vi "PH_ImageCoG_Plotter.ProcCases.vi"(0 "i ref in":refnum<vi>, 1 "selector":string, 2 "data":T1, 3 "call cluster":T2={"Object"="", "Selector"="", "CallType"=enum."synchronous", "Async Object"="", "Async Selector"="", "Data Descriptor"="", "Data"=[], "Error #"=0, "Expire"=0}, 5 "error in":errorcluster) -> (14 "i ref out":refnum<vi>, 17 "answer cluster":T2={"Object"="", "Selector"="", "CallType"=enum."synchronous", "Async Object"="", "Async Selector"="", "Data Descriptor"="", "Data"=[], "Error #"=0, "Expire"=0}, 19 "error out":errorcluster)   [LabVIEW 2014, in "PH_ImageCoG_Plotter.lvlib"]
doc: "This method is called by a process from within the default case in the event loop. The methods of a class that are linked to events will be called from THIS method. Add your code here."
uses:
  PH_ImageCoG_Plotter.lvlib
  CS_Core/CSSystem/CoreDefs/CoreDefs.call_type.ctl
  CS_Core/BaseProcess/BaseProcess.descriptor string definition.ctl
  CS_Core/CSSystem/CoreDefs/CoreDefs.rawDataType.ctl
  CS_Core/CSSystem/CoreLib/CoreLib.byte array 2 int.vi
  CS_Core/CSSystem/CoreLib/CoreLib.string 2 byte array.vi
  CS_Core/CSSystem/CoreLib/CoreLib.byte array 2 short.vi
  CS_Core/CSSystem/CoreLib/CoreLib.byte array 2 string.vi
  CS_Core/CSSystem/CoreLib/CoreLib.lvlib
  CS_Core/BaseProcess/BaseProcess.lvlib
  CS_Core/CAEObj/CAEObj.lvlib
  PH_Basics/PH_Img_BaseClass/PH_Img_BaseClass.lvlib
  PH_Basics/PH_Cam_BaseClass/PH_Cam_BaseClass.lvlib
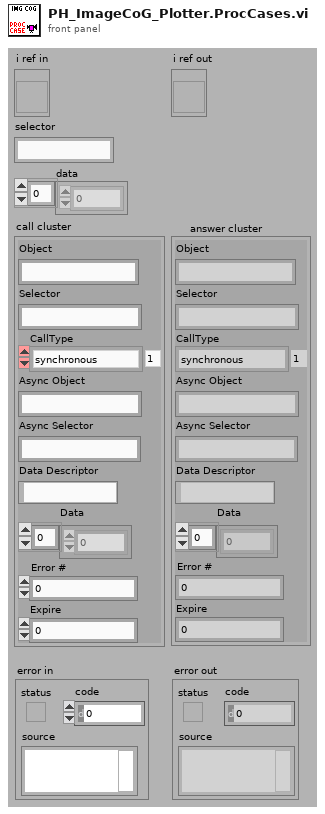
[diagram p1: front panel]
types:
  T1 = typedef "CoreDefs.rawDataType.ctl" = i8[]
  T2 = typedef "CoreDefs.call_type.ctl" = cluster{"Object":string, "Selector":string, "CallType":enum16{"simple", "synchronous", "asynchronous"}, "Async Object":string, "Async Selector":string, "Data Descriptor":T3, "Data":T1, "Error #":i32, "Expire":u32}
  T3 = typedef "BaseProcess.lvlib/BaseProcess.descriptor string definition.ctl" = string
  T4 = typedef "PH_ImageCoG_Plotter.lvlib/PH_ImageCoG_Plotter.i attribute.ctl" = cluster{"GUI Refs":cluster{"Delete":refnum<vi>, "Calibration status":refnum<vi>, "BI subtracted":refnum<vi>, "calc Beam Anal":refnum<vi>, "CoG - x":refnum<vi>, "CoG - y":refnum<vi>, "Type":refnum<vi>, "Center":refnum<vi>, "exp - X":refnum<vi>, "exp - Y":refnum<vi>, "Delta - X":refnum<vi>, "Delta - Y":refnum<vi>, "Available Cams":refnum<vi>, "CoG X":refnum<vi>, "CoG Y":refnum<vi>, "Delta X":refnum<vi>, "Delta Y":refnum<vi>, "Export Data":refnum<vi>, "Calibration data":refnum<vi>}, "Calibration":cluster{"Status":T5, "Calibration data":T6, "Calibration Data File":path}, "Beam Analysis":cluster{"on":bool, "exp - X":i32, "exp - Y":i32, "Type":bool, "Data":cluster{"current time":timestamp, "CoG-x":dbl, "CoG-y":dbl, "Delta-x":dbl, "Delta-y":dbl}[], "Datasets strored":i32, "Dataarray Size":i32}, "Cam instances":string[], "DIM Service Events":T7[], "Images":cluster{"Background":T9, "OP":T9, "GUI":T9}}
  T5 = typedef "PH_StatusHandler.lvlib/PH_StatusHandler.Status.ctl" = i16
  T6 = typedef "PH_ImageCalibrator.lvlib/PH_ImageCalibrator.Calibration Data.ctl" = cluster{"Date":string, "Time":string, "Cam Settings":cluster{"Cam ID":string, "Gain":dbl, "Brightness":dbl, "Shutter":dbl, "Cam Error":bool, "Mode":i32}, "Background Image":cluster{"Image":dbl[][], "Image Error":bool}, "Linear Calibration":cluster{"Calibration Factor":dbl, "not mm or mrad":bool}, "Energy Calibration":cluster{"Calibration Factor":dbl, "no mJ":bool}}
  T7 = typedef "BaseProcess.lvlib/BaseProcess.event definition.ctl" = cluster{"CAEEvtDef":T8, "Data Descriptor":T3}
  T8 = typedef "CAEObj.lvlib/CAEObj.event definition.ctl" = cluster{"URL":string, "enable":bool, "ignoreResID":bool}
  T9 = typedef "IMAQ Image.ctl" = refnum<image>
  T10 = typedef "PH_Cam_BaseClass.lvlib/PH_Cam_BaseClass.Settings.ctl" = cluster{"Cam ID":string, "Gain":dbl, "Brightness":dbl, "Shutter":dbl, "Mode":i32}
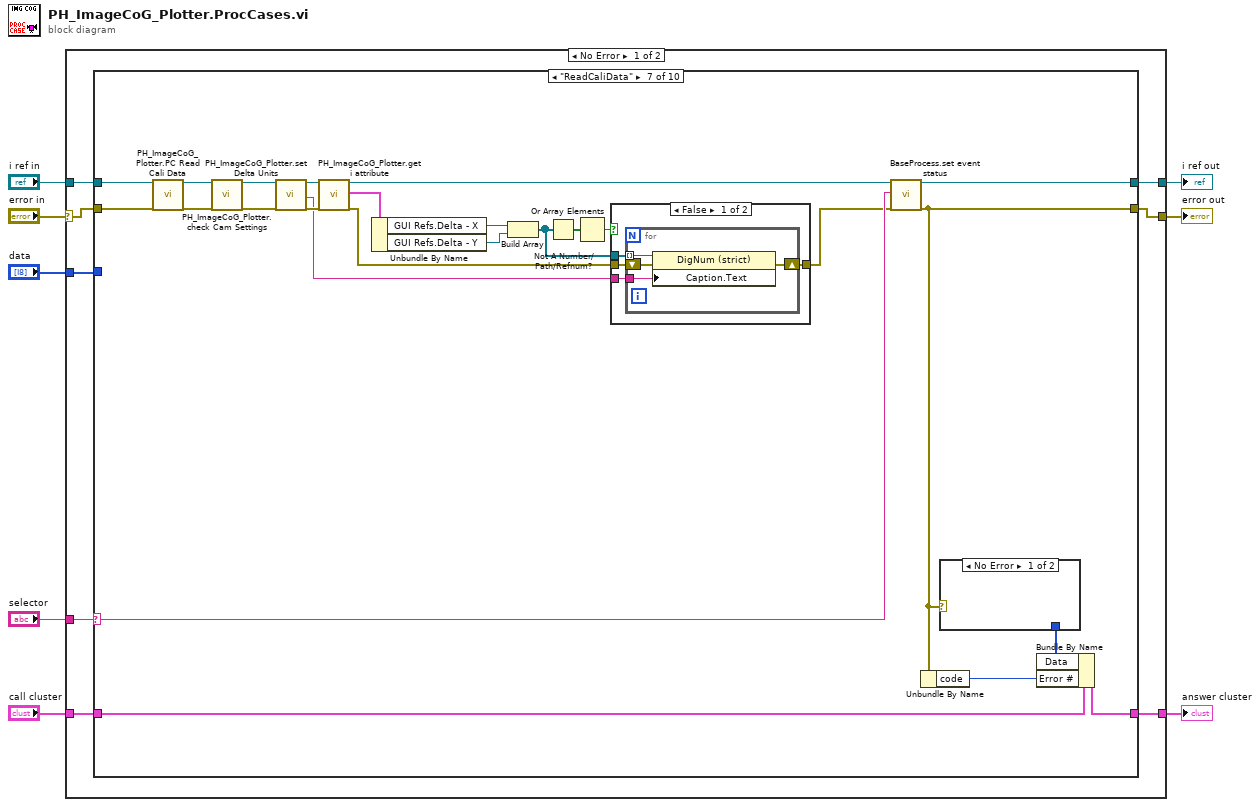
[diagram p0: block diagram]
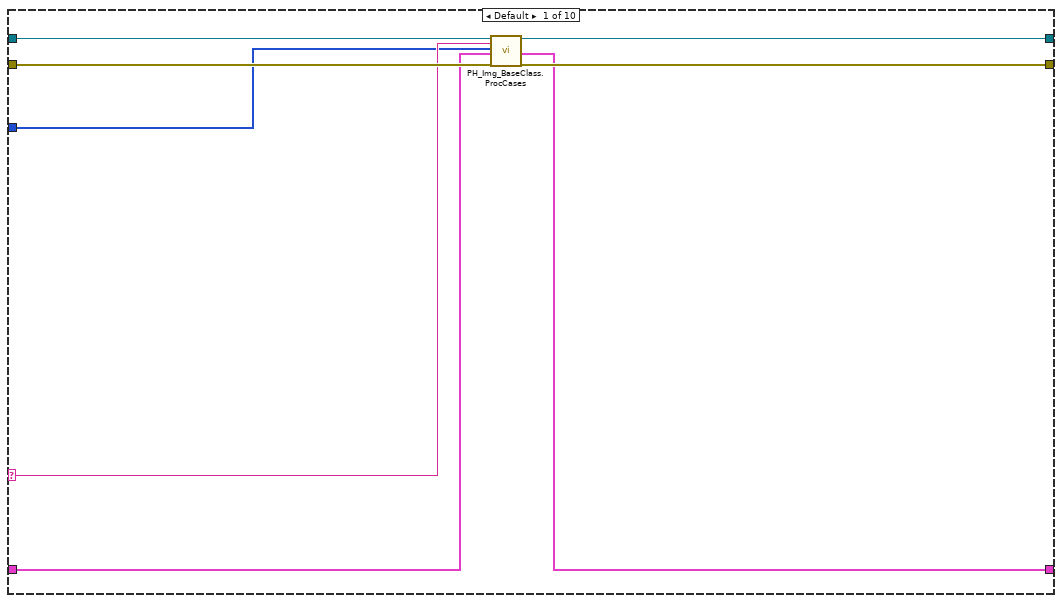
[diagram p2: hidden frame]
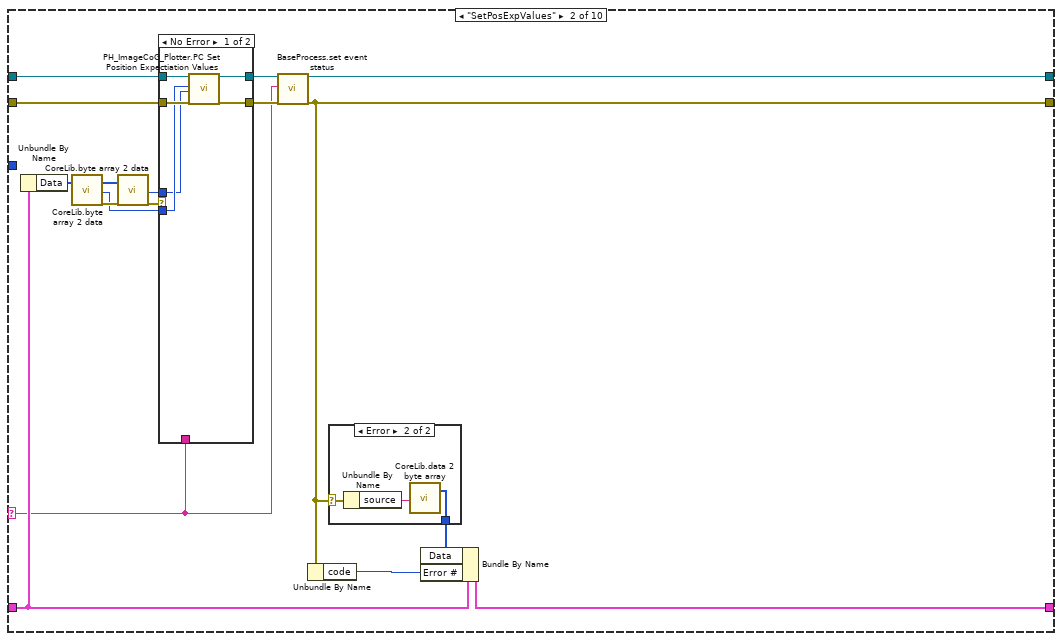
[diagram p3: hidden frame]
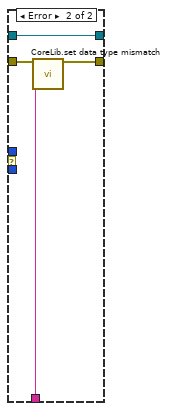
[diagram p5: hidden frame]
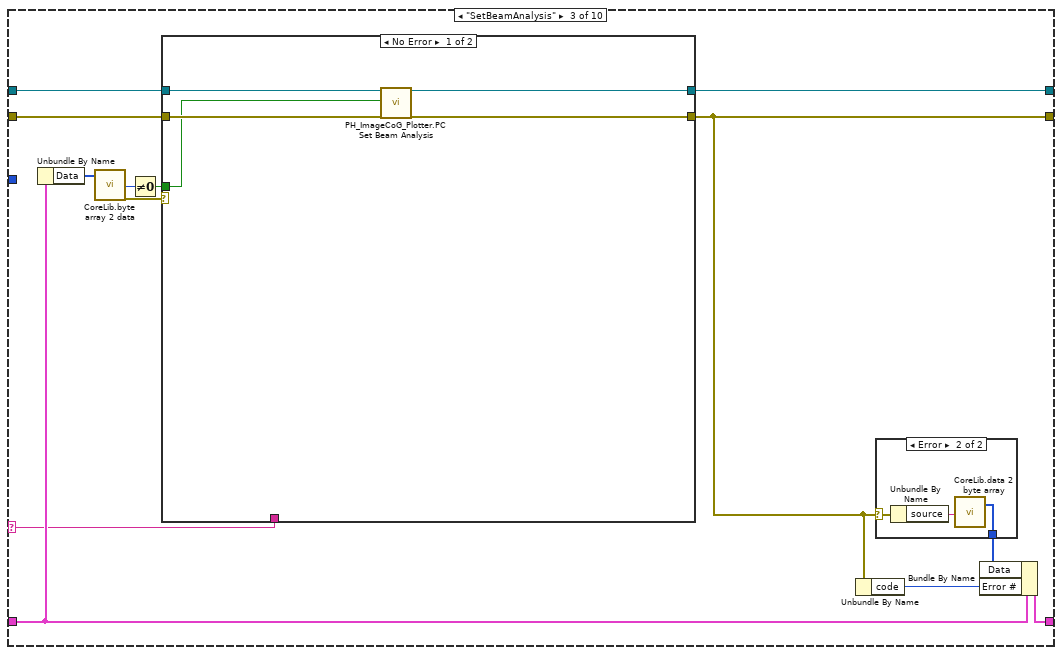
[diagram p6: hidden frame]
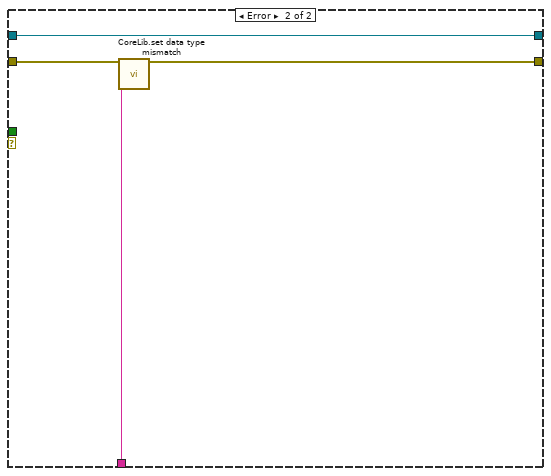
[diagram p7: hidden frame]
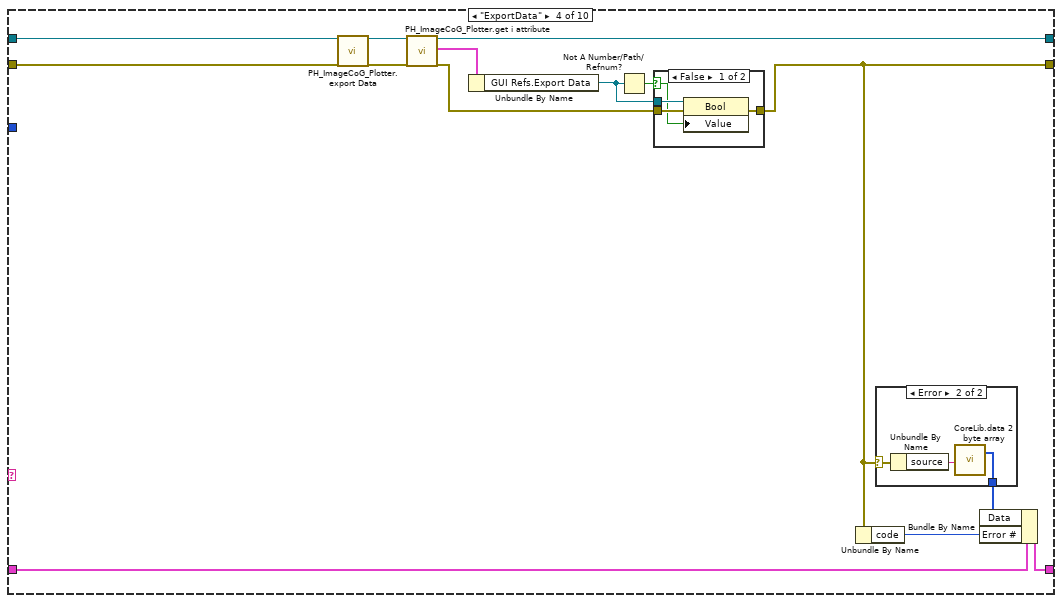
[diagram p9: hidden frame]
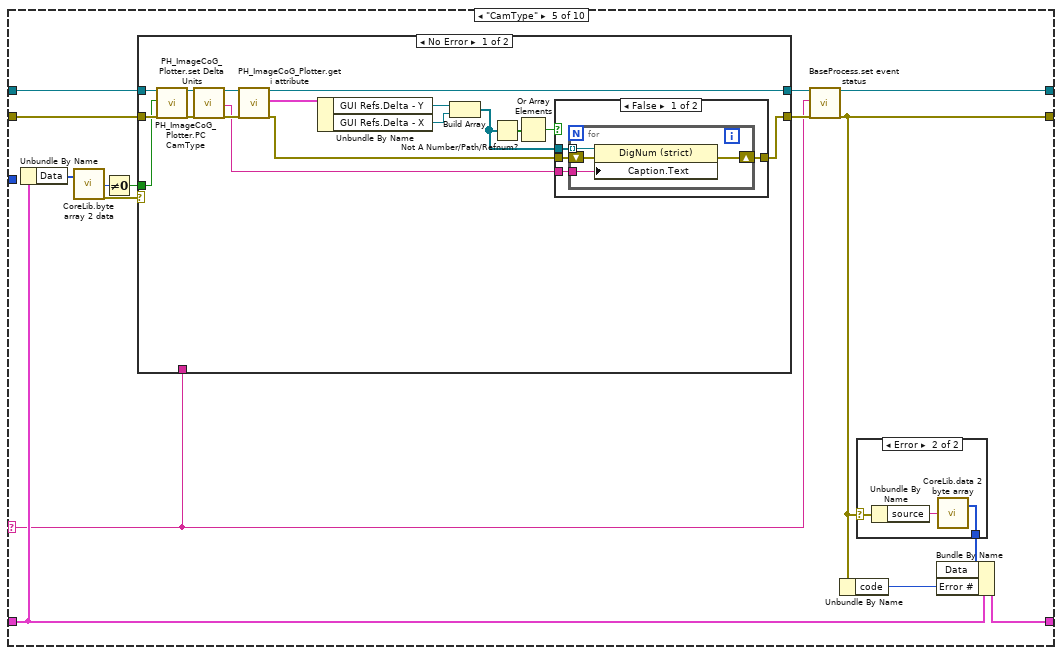
[diagram p12: hidden frame]
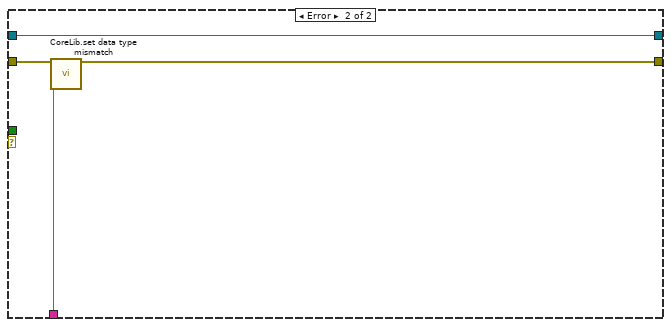
[diagram p15: hidden frame]
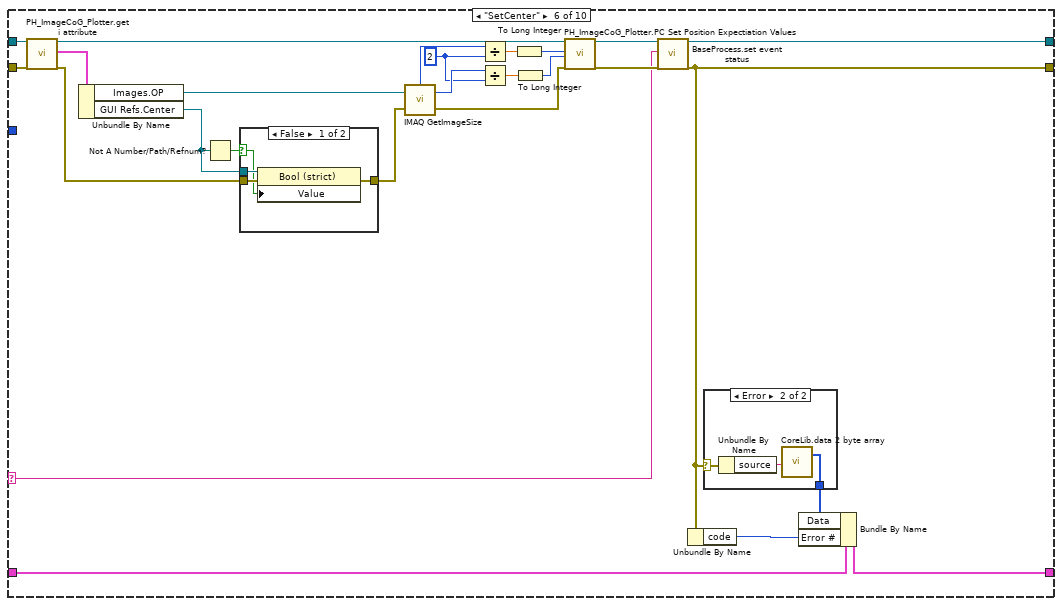
[diagram p16: hidden frame]
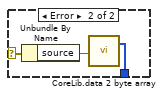
[diagram p20: hidden frame]
diagram:
  n1 = case shown="No Error" "error in" {
    selector: "error in" -> [w9 w336]
    tunnel: "selector" -> [w16 _]
    tunnel: [w15 w335] -> w7
    tunnel: "call cluster" -> [w14 w335]
    tunnel: "i ref in" -> [w13 w337]
    tunnel: [w12 w337] -> w5
    tunnel: [w11 w336] -> w4
    tunnel: "data" -> [w10 _]
    frame No Error {
      n2 = case shown="\"ReadCaliData\"" w16 {
        selector: w16 -> [w19 w33 w55 _ w108 w169 w204 w235 w243 w275]
        tunnel: w10 -> [w17 _ _ _ _ _ _ _ _ w274]
        tunnel: w13 -> [w18 w41 w58 w89 w116 w167 w202 w231 w246 w273]
        tunnel: [w24 w32 w57 w86 w107 w168 w203 w234 w253 w281] -> w12
        tunnel: w14 -> [w20 w38 w60 w90 w113 w174 w207 w238 w248 w279]
        tunnel: [w21 w37 w66 w92 w112 w173 w206 w237 w255 w283] -> w15
        tunnel: w9 -> [w23 w40 w59 w88 w115 w165 w201 w232 w247 w278]
        tunnel: [w22 w34 w56 w82 w109 w170 w205 w236 w254 w282] -> w11
        frame Default {
          n3 = call "PH_Img_BaseClass.ProcCases.vi"("i ref in"=w18, "selector"=w19, "Data"=w17, "call cluster"=w20, "error in (no error)"=w23) -> ("i ref out"=w24:refnum<vi>, "answer cluster"=w21:T2, "error out"=w22:errorcluster)  [unwired: 12 in]
        }
        frame "SetPosExpValues" {
          n4 = Unbundle By Name(w38) -> ("Data"=w26:T1)
          n5 = call-poly "CoreLib.byte array 2 data.vi"("byteArray"=w26) -> ("byteArray out"=w31:T1, "i32"=w29:i32, "error out"=w30:errorcluster)  [unwired: 16 in]
          n6 = call-poly "CoreLib.byte array 2 data.vi"("byteArray"=w31, "error in (no error)"=w30) -> ("i32"=w28:i32, "error out"=w27:errorcluster)  [unwired: 15 in, 1 out]
          n7 = case shown="No Error" w27 {
            tunnel: [w49 w54] -> w36
            tunnel: w41 -> [w50 w54]
            tunnel: w40 -> [w48 w53]
            tunnel: [w47 w52] -> w35
            tunnel: w29 -> [w46 _]
            tunnel: w33 -> [_ w51]
            tunnel: w28 -> [w45 _]
            frame No Error {
              n8 = call "PH_ImageCoG_Plotter.PC Set Position Expectiation Values.vi"("i ref in"=w50, "expected X"=w46, "expected Y"=w45, "error in (no error)"=w48) -> ("i ref out"=w49:refnum<vi>, "error out"=w47:errorcluster)  [unwired: 14 in]
            }
            frame Error {
              n9 = call "CoreLib.set data type mismatch.vi"("error in (no error)"=w53, "error source"=w51) -> ("error out"=w52:errorcluster)  [unwired: 17 in]
            }
          }
          n10 = call "BaseProcess.set event status.vi"("i ref in"=w36, "EventStatus"=w33, "error in (no error)"=w35) -> ("i ref out"=w32:refnum<vi>, "error out"=w34:errorcluster)  [unwired: 14 in, 1 out]
          n11 = Unbundle By Name(w34) -> ("code"=w39:i32)
          n12 = case shown="Error" w34 {
            selector: w34 -> [_ w44]
            tunnel: [_ w42] -> w25
            frame No Error {
            }
            frame Error {
              n13 = Unbundle By Name(w44) -> ("source"=w43:string)
              n14 = call-poly "CoreLib.data 2 byte array.vi"("string"=w43) -> ("byteArray out"=w42:T1)  [unwired: 18 in]
            }
          }
          n15 = Bundle By Name(cluster=w38, "Data"=w25, "Error #"=w39) -> (w37:T2)
        }
        frame "SetBeamAnalysis" {
          n16 = Unbundle By Name(w60) -> ("Data"=w63:T1)
          n17 = call-poly "CoreLib.byte array 2 data.vi"("byteArray"=w63) -> ("i16"=w64:i16, "error out"=w61:errorcluster)  [unwired: 16 in, 1 out]
          n18 = Not Equal To 0?(x=w64) -> (x != 0?=w62:bool)
          n19 = case shown="No Error" w61 {
            tunnel: [w70 w76] -> w57
            tunnel: w58 -> [w72 w76]
            tunnel: w59 -> [w71 w75]
            tunnel: [w69 w74] -> w56
            tunnel: w55 -> [_ w73]
            tunnel: w62 -> [w68 _]
            frame No Error {
              n20 = call "PH_ImageCoG_Plotter.PC Set Beam Analysis.vi"("i ref in"=w72, "On / Off"=w68, "error in (no error)"=w71) -> ("i ref out"=w70:refnum<vi>, "error out"=w69:errorcluster)  [unwired: 15 in]
            }
            frame Error {
              n21 = call "CoreLib.set data type mismatch.vi"("error in (no error)"=w75, "error source"=w73) -> ("error out"=w74:errorcluster)  [unwired: 17 in]
            }
          }
          n22 = Unbundle By Name(w56) -> ("code"=w67:i32)
          n23 = case shown="Error" w56 {
            selector: w56 -> [_ w79]
            tunnel: [_ w77] -> w65
            frame No Error {
            }
            frame Error {
              n24 = Unbundle By Name(w79) -> ("source"=w78:string)
              n25 = call-poly "CoreLib.data 2 byte array.vi"("string"=w78) -> ("byteArray out"=w77:T1)  [unwired: 18 in]
            }
          }
          n26 = Bundle By Name(cluster=w60, "Data"=w65, "Error #"=w67) -> (w66:T2)
        }
        frame "ExportData" {
          n27 = call "PH_ImageCoG_Plotter.export Data.vi"("i ref in"=w89, "error in (no error)"=w88) -> ("i ref out"=w87:refnum<vi>, "error out"=w85:errorcluster)  [unwired: 16 in]
          n28 = call "PH_ImageCoG_Plotter.get i attribute.vi"("i ref in"=w87, "error in (no error)"=w85) -> ("i ref out"=w86:refnum<vi>, "i attribute"=w84:T4, "error out"=w83:errorcluster)  [unwired: 15 in]
          n29 = Unbundle By Name(w84) -> ("GUI Refs.Export Data"=w80:refnum<vi>)
          n30 = Not A Number/Path/Refnum?(number/path/refnum=w80) -> (NaN/Path/Refnum?=w81:bool)
          n31 = case shown="False" w81 {
            selector: w81 -> [w94 _]
            tunnel: w80 -> [w97 _]
            tunnel: w83 -> [w96 w98]
            tunnel: [w95 w98] -> w82
            frame False {
              n32 = property class="Bool"(reference=w97, error in=w96, "Value"=w94) -> (error out=w95:errorcluster)  [unwired: 1 out]
            }
            frame True {
            }
          }
          n33 = Unbundle By Name(w82) -> ("code"=w93:i32)
          n34 = case shown="Error" w82 {
            selector: w82 -> [_ w101]
            tunnel: [_ w99] -> w91
            frame No Error {
            }
            frame Error {
              n35 = Unbundle By Name(w101) -> ("source"=w100:string)
              n36 = call-poly "CoreLib.data 2 byte array.vi"("string"=w100) -> ("byteArray out"=w99:T1)  [unwired: 18 in]
            }
          }
          n37 = Bundle By Name(cluster=w90, "Data"=w91, "Error #"=w93) -> (w92:T2)
        }
        frame "CamType" {
          n38 = Unbundle By Name(w113) -> ("Data"=w105:T1)
          n39 = call-poly "CoreLib.byte array 2 data.vi"("byteArray"=w105) -> ("i16"=w106:i16, "error out"=w103:errorcluster)  [unwired: 16 in, 1 out]
          n40 = Not Equal To 0?(x=w106) -> (x != 0?=w104:bool)
          n41 = case shown="No Error" w103 {
            tunnel: [w121 w149] -> w111
            tunnel: w116 -> [w136 w149]
            tunnel: w115 -> [w135 w148]
            tunnel: [w123 w147] -> w110
            tunnel: w108 -> [_ w146]
            tunnel: w104 -> [w134 _]
            frame No Error {
              n42 = call "PH_ImageCoG_Plotter.PC CamType.vi"("i ref in"=w136, "Nearfield/Farfield"=w134, "error in (no error)"=w135) -> ("i ref out"=w132:refnum<vi>, "error out"=w133:errorcluster)  [unwired: 15 in]
              n43 = call "PH_ImageCoG_Plotter.set Delta Units.vi"("i ref in"=w132, "error in (no error)"=w133) -> ("i ref out"=w122:refnum<vi>, "Unit"=w120:string, "error out"=w124:errorcluster)  [unwired: 15 in]
              n44 = call "PH_ImageCoG_Plotter.get i attribute.vi"("i ref in"=w122, "error in (no error)"=w124) -> ("i ref out"=w121:refnum<vi>, "i attribute"=w125:T4, "error out"=w131:errorcluster)  [unwired: 15 in]
              n45 = Unbundle By Name(w125) -> ("GUI Refs.Delta - Y"=w129:refnum<vi>, "GUI Refs.Delta - X"=w128:refnum<vi>)
              n46 = Build Array(w129, w128) -> (w127:refnum<vi>[])
              n47 = Not A Number/Path/Refnum?(number/path/refnum=w127) -> (NaN/Path/Refnum?=w130:bool[])
              n48 = Or Array Elements(Boolean array=w130) -> (logical OR=w126:bool)
              n49 = case shown="False" w126 {
                tunnel: w127 -> [w140 _]
                tunnel: w120 -> [w139 _]
                tunnel: w131 -> [w138 w145]
                tunnel: [w137 w145] -> w123
                frame False {
                  n50 = for {
                    tunnel: w140 -> [w144] mode=indexing
                    tunnel: w139 -> [w143]
                    shift-right: [w141] -> w137
                    shift-left: w138 -> [w142]
                    n51 = property class="DigNum (strict)"(reference=w144, error in=w142, "Caption.Text"=w143) -> (error out=w141:errorcluster)  [unwired: 1 out]
                  }
                }
                frame True {
                }
              }
            }
            frame Error {
              n52 = call "CoreLib.set data type mismatch.vi"("error in (no error)"=w148, "error source"=w146) -> ("error out"=w147:errorcluster)  [unwired: 17 in]
            }
          }
          n53 = call "BaseProcess.set event status.vi"("i ref in"=w111, "EventStatus"=w108, "error in (no error)"=w110) -> ("i ref out"=w107:refnum<vi>, "error out"=w109:errorcluster)  [unwired: 14 in, 1 out]
          n54 = Unbundle By Name(w109) -> ("code"=w114:i32)
          n55 = case shown="Error" w109 {
            selector: w109 -> [_ w119]
            tunnel: [_ w117] -> w102
            frame No Error {
            }
            frame Error {
              n56 = Unbundle By Name(w119) -> ("source"=w118:string)
              n57 = call-poly "CoreLib.data 2 byte array.vi"("string"=w118) -> ("byteArray out"=w117:T1)  [unwired: 18 in]
            }
          }
          n58 = Bundle By Name(cluster=w113, "Data"=w102, "Error #"=w114) -> (w112:T2)
        }
        frame "SetCenter" {
          w160 = 2 ("y")
          n59 = call "PH_ImageCoG_Plotter.get i attribute.vi"("i ref in"=w167, "error in (no error)"=w165) -> ("i ref out"=w166:refnum<vi>, "i attribute"=w164:T4, "error out"=w154:errorcluster)  [unwired: 15 in]
          n60 = Unbundle By Name(w164) -> ("Images.OP"=w150:T9, "GUI Refs.Center"=w152:refnum<vi>)
          n61 = Not A Number/Path/Refnum?(number/path/refnum=w152) -> (NaN/Path/Refnum?=w153:bool)
          n62 = case shown="False" w153 {
            selector: w153 -> [w176 _]
            tunnel: [w179 w180] -> w155
            tunnel: w154 -> [w178 w180]
            tunnel: w152 -> [w177 _]
            frame False {
              n63 = property class="Bool (strict)"(reference=w177, error in=w178, "Value"=w176) -> (error out=w179:errorcluster)  [unwired: 1 out]
            }
            frame True {
            }
          }
          n64 = call "IMAQ GetImageSize"("Image"=w150, "error in (no error)"=w155) -> ("Y Resolution"=w161:i32, "X Resolution"=w162:i32, "error out"=w163:errorcluster)  [unwired: 2 in]
          n65 = Divide(x=w162, y=w160) -> (x/y=w159:dbl)
          n66 = Divide(x=w161, y=w160) -> (x/y=w158:dbl)
          n67 = To Long Integer(number=w159) -> (32bit integer=w156:i32)
          n68 = To Long Integer(number=w158) -> (32bit integer=w157:i32)
          n69 = call "PH_ImageCoG_Plotter.PC Set Position Expectiation Values.vi"("i ref in"=w166, "expected X"=w156, "expected Y"=w157, "error in (no error)"=w163) -> ("i ref out"=w172:refnum<vi>, "error out"=w171:errorcluster)  [unwired: 14 in]
          n70 = call "BaseProcess.set event status.vi"("i ref in"=w172, "EventStatus"=w169, "error in (no error)"=w171) -> ("i ref out"=w168:refnum<vi>, "error out"=w170:errorcluster)  [unwired: 14 in, 1 out]
          n71 = Unbundle By Name(w170) -> ("code"=w175:i32)
          n72 = case shown="Error" w170 {
            selector: w170 -> [_ w183]
            tunnel: [_ w181] -> w151
            frame No Error {
            }
            frame Error {
              n73 = Unbundle By Name(w183) -> ("source"=w182:string)
              n74 = call-poly "CoreLib.data 2 byte array.vi"("string"=w182) -> ("byteArray out"=w181:T1)  [unwired: 18 in]
            }
          }
          n75 = Bundle By Name(cluster=w174, "Data"=w151, "Error #"=w175) -> (w173:T2)
        }
        frame "ReadCaliData" {
          n76 = call "PH_ImageCoG_Plotter.PC Read Cali Data.vi"("i ref in"=w202, "error in (no error)"=w201) -> ("i ref out"=w187:refnum<vi>, "error out"=w185:errorcluster)  [unwired: 16 in]
          n77 = call "PH_ImageCoG_Plotter.check Cam Settings.vi"("i ref in"=w187, "error out"=w185) -> ("i ref out"=w186:refnum<vi>, "error out"=w184:errorcluster)  [unwired: 16 in]
          n78 = call "PH_ImageCoG_Plotter.set Delta Units.vi"("i ref in"=w186, "error in (no error)"=w184) -> ("i ref out"=w199:refnum<vi>, "Unit"=w188:string, "error out"=w197:errorcluster)  [unwired: 15 in]
          n79 = call "PH_ImageCoG_Plotter.get i attribute.vi"("i ref in"=w199, "error in (no error)"=w197) -> ("i ref out"=w198:refnum<vi>, "i attribute"=w194:T4, "error out"=w196:errorcluster)  [unwired: 15 in]
          n80 = Unbundle By Name(w194) -> ("GUI Refs.Delta - X"=w193:refnum<vi>, "GUI Refs.Delta - Y"=w192:refnum<vi>)
          n81 = Build Array(w193, w192) -> (w191:refnum<vi>[])
          n82 = Not A Number/Path/Refnum?(number/path/refnum=w191) -> (NaN/Path/Refnum?=w190:bool[])
          n83 = Or Array Elements(Boolean array=w190) -> (logical OR=w189:bool)
          n84 = case shown="False" w189 {
            tunnel: w196 -> [w212 w217]
            tunnel: [w211 w217] -> w195
            tunnel: w191 -> [w210 _]
            tunnel: w188 -> [w209 _]
            frame False {
              n85 = for {
                shift-right: [w215] -> w211
                shift-left: w212 -> [w216]
                tunnel: w210 -> [w214] mode=indexing
                tunnel: w209 -> [w213]
                n86 = property class="DigNum (strict)"(reference=w214, error in=w216, "Caption.Text"=w213) -> (error out=w215:errorcluster)  [unwired: 1 out]
              }
            }
            frame True {
            }
          }
          n87 = call "BaseProcess.set event status.vi"("i ref in"=w198, "EventStatus"=w204, "error in (no error)"=w195) -> ("i ref out"=w203:refnum<vi>, "error out"=w205:errorcluster)  [unwired: 14 in, 1 out]
          n88 = Unbundle By Name(w205) -> ("code"=w208:i32)
          n89 = case shown="No Error" w205 {
            selector: w205 -> [_ w220]
            tunnel: [_ w218] -> w200
            frame No Error {
            }
            frame Error {
              n90 = Unbundle By Name(w220) -> ("source"=w219:string)
              n91 = call-poly "CoreLib.data 2 byte array.vi"("string"=w219) -> ("byteArray out"=w218:T1)  [unwired: 18 in]
            }
          }
          n92 = Bundle By Name(cluster=w207, "Data"=w200, "Error #"=w208) -> (w206:T2)
        }
        frame "getCamInstances" {
          n93 = call "PH_ImageCoG_Plotter.get Cam instances.vi"("i ref in"=w231, "error in"=w232) -> ("i ref out"=w224:refnum<vi>, "error out"=w222:errorcluster)  [unwired: 16 in]
          n94 = call "PH_ImageCoG_Plotter.get i attribute.vi"("i ref in"=w224, "error in (no error)"=w222) -> ("i ref out"=w225:refnum<vi>, "i attribute"=w229:T4, "error out"=w230:errorcluster)  [unwired: 15 in]
          n95 = Unbundle By Name(w229) -> ("Cam instances"=w228:string[])
          n96 = Index Array(array=w228, index=0) -> (element=w226:string)
          n97 = call "PH_ImageCoG_Plotter.PC set selected Cam.vi"("VI in"=w225, "Camera to select"=w226, "error in (no error)"=w230) -> ("VI out"=w223:refnum<vi>, "error out"=w221:errorcluster)  [unwired: 15 in]
          n98 = call "BaseProcess.set event status.vi"("i ref in"=w223, "EventStatus"=w235, "error in (no error)"=w221) -> ("i ref out"=w234:refnum<vi>, "error out"=w236:errorcluster)  [unwired: 14 in, 1 out]
          n99 = Unbundle By Name(w236) -> ("code"=w239:i32)
          n100 = case shown="No Error" w236 {
            selector: w236 -> [_ w242]
            tunnel: [_ w240] -> w233
            frame No Error {
            }
            frame Error {
              n101 = Unbundle By Name(w242) -> ("source"=w241:string)
              n102 = call-poly "CoreLib.data 2 byte array.vi"("string"=w241) -> ("byteArray out"=w240:T1)  [unwired: 18 in]
            }
          }
          n103 = Bundle By Name(cluster=w238, "Data"=w233, "Error #"=w239) -> (w237:T2)
        }
        frame "SelectCam" {
          n104 = Unbundle By Name(w248) -> ("Data"=w251:T1)
          n105 = call-poly "CoreLib.byte array 2 data.vi"("byteArray"=w251) -> ("string"=w250:string, "error out"=w249:errorcluster)  [unwired: 16 in, 1 out]
          n106 = case shown="No Error" w249 {
            tunnel: w246 -> [w260 w263]
            tunnel: [w259 w263] -> w245
            tunnel: w247 -> [w261 w265]
            tunnel: [w258 w264] -> w244
            tunnel: w243 -> [_ w262]
            tunnel: w250 -> [w257 _]
            frame No Error {
              n107 = call "PH_ImageCoG_Plotter.PC set selected Cam.vi"("VI in"=w260, "Camera to select"=w257, "error in (no error)"=w261) -> ("VI out"=w259:refnum<vi>, "error out"=w258:errorcluster)  [unwired: 15 in]
            }
            frame Error {
              n108 = call "CoreLib.set data type mismatch.vi"("error in (no error)"=w265, "error source"=w262) -> ("error out"=w264:errorcluster)  [unwired: 17 in]
            }
          }
          n109 = call "BaseProcess.set event status.vi"("i ref in"=w245, "EventStatus"=w243, "error in (no error)"=w244) -> ("i ref out"=w253:refnum<vi>, "error out"=w254:errorcluster)  [unwired: 14 in, 1 out]
          n110 = Unbundle By Name(w254) -> ("code"=w256:i32)
          n111 = case shown="Error" w254 {
            selector: w254 -> [_ w268]
            tunnel: [_ w266] -> w252
            frame No Error {
            }
            frame Error {
              n112 = Unbundle By Name(w268) -> ("source"=w267:string)
              n113 = call-poly "CoreLib.data 2 byte array.vi"("string"=w267) -> ("byteArray out"=w266:T1)  [unwired: 18 in]
            }
          }
          n114 = Bundle By Name(cluster=w248, "Data"=w252, "Error #"=w256) -> (w255:T2)
        }
        frame "_Settings" {
          n115 = call "CAEObj.unfold trend data.vi"("i ref in"=w273, "raw trend data"=w274) -> ("no link"=w269:bool, "data"=w270:i8[], "typeDescriptor"=w271:string, "error out"=w272:errorcluster)  [unwired: 9 in, 5 out]
          n116 = case shown="No Error" w272 {
            tunnel: w273 -> [w306 w331]
            tunnel: [w292 w331] -> w277
            tunnel: w278 -> [w308 w330]
            tunnel: [w290 w330] -> w276
            tunnel: w271 -> [w311 _]
            tunnel: w270 -> [w310 _]
            tunnel: w269 -> [w287 _]
            frame No Error {
              n117 = case shown="\"C\", \"C:N\"" w311 {
                tunnel: w310 -> [_ w329]
                tunnel: [string[] [] ("Array") w327] -> w309
                frame Default {
                }
                frame "C", "C:N" {
                  n118 = Type Cast(x=w329) -> (*(type *) &x=w328:string)  [unwired: 1 in]
                  n119 = call "CoreLib.stringToStringArray.vi"("String"=w328) -> ("Array"=w327:string[])
                }
              }
              n120 = call "PH_Cam_BaseClass.Setting Unpacker.vi"("Cam Settings Array"=w309, "error in (no error)"=w308) -> ("Cam Settings"=w303:T10, "error out"=w307:errorcluster)  [unwired: 15 in, 1 out]
              n121 = call "PH_ImageCoG_Plotter.get Cam Settings.vi"("i ref in"=w306, "Cam Settings"=w303, "Cam Info Failure"=w287, "error in (no error)"=w307) -> ("i ref out"=w305:refnum<vi>, "error out"=w304:errorcluster)  [unwired: 14 in]
              n122 = call "PH_ImageCoG_Plotter.check Cam Settings.vi"("i ref in"=w305, "error out"=w304) -> ("i ref out"=w293:refnum<vi>, "error out"=w291:errorcluster)  [unwired: 16 in]
              n123 = call "PH_ImageCoG_Plotter.set Delta Units.vi"("i ref in"=w293, "error in (no error)"=w291) -> ("i ref out"=w302:refnum<vi>, "Unit"=w294:string, "error out"=w301:errorcluster)  [unwired: 15 in]
              n124 = call "PH_ImageCoG_Plotter.get i attribute.vi"("i ref in"=w302, "error in (no error)"=w301) -> ("i ref out"=w292:refnum<vi>, "i attribute"=w300:T4, "error out"=w286:errorcluster)  [unwired: 15 in]
              n125 = Unbundle By Name(w300) -> ("GUI Refs.Available Cams"=w288:refnum<vi>, "GUI Refs.Delta - X"=w299:refnum<vi>, "GUI Refs.Delta - Y"=w298:refnum<vi>)
              n126 = Build Array(w299, w298) -> (w297:refnum<vi>[])
              n127 = Not A Number/Path/Refnum?(number/path/refnum=w297) -> (NaN/Path/Refnum?=w296:bool[])
              n128 = Not A Number/Path/Refnum?(number/path/refnum=w288) -> (NaN/Path/Refnum?=w289:bool)
              n129 = Or Array Elements(Boolean array=w296) -> (logical OR=w295:bool)
              n130 = case shown="False" w289 {
                tunnel: w286 -> [w315 w316]
                tunnel: [w314 w316] -> w285
                tunnel: w288 -> [w313 _]
                tunnel: w287 -> [w312 _]
                frame False {
                  n131 = property class="Ring (strict)"(reference=w313, error in=w315, "Blinking"=w312) -> (error out=w314:errorcluster)  [unwired: 1 out]
                }
                frame True {
                }
              }
              n132 = case shown="False" w295 {
                tunnel: w285 -> [w320 w325]
                tunnel: [w319 w325] -> w290
                tunnel: w297 -> [w318 _]
                tunnel: w294 -> [w317 _]
                frame False {
                  n133 = for {
                    shift-right: [w323] -> w319
                    shift-left: w320 -> [w324]
                    tunnel: w318 -> [w322] mode=indexing
                    tunnel: w317 -> [w321]
                    n134 = property class="DigNum (strict)"(reference=w322, error in=w324, "Caption.Text"=w321) -> (error out=w323:errorcluster)  [unwired: 1 out]
                  }
                }
                frame True {
                }
              }
            }
            frame Error {
            }
          }
          n135 = call "BaseProcess.set event status.vi"("i ref in"=w277, "EventStatus"=w275, "error in (no error)"=w276) -> ("i ref out"=w281:refnum<vi>, "error out"=w282:errorcluster)  [unwired: 14 in, 1 out]
          n136 = Unbundle By Name(w282) -> ("code"=w284:i32)
          n137 = case shown="Error" w282 {
            selector: w282 -> [_ w334]
            tunnel: [_ w332] -> w280
            frame No Error {
            }
            frame Error {
              n138 = Unbundle By Name(w334) -> ("source"=w333:string)
              n139 = call-poly "CoreLib.data 2 byte array.vi"("string"=w333) -> ("byteArray out"=w332:T1)  [unwired: 18 in]
            }
          }
          n140 = Bundle By Name(cluster=w279, "Data"=w280, "Error #"=w284) -> (w283:T2)
        }
      }
    }
    frame Error {
    }
  }
  "answer cluster" <- w7
  "i ref out" <- w5
  "error out" <- w4
